vi "Test Event Registration.vi"() -> ()   [LabVIEW 2019]
panel:
  out "string 1":string
  in  "String Control":string
  in  "stop":bool
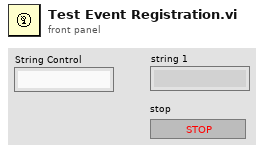
[diagram p1: front panel]
types:
  T1 = cluster{"string 2":refnum<user-event>, "string 3":refnum<user-event>}
  T2 = cluster{"Event Registration Refnum":refnum<event-registration>, "Event Registration Refnum":refnum<event-registration>}
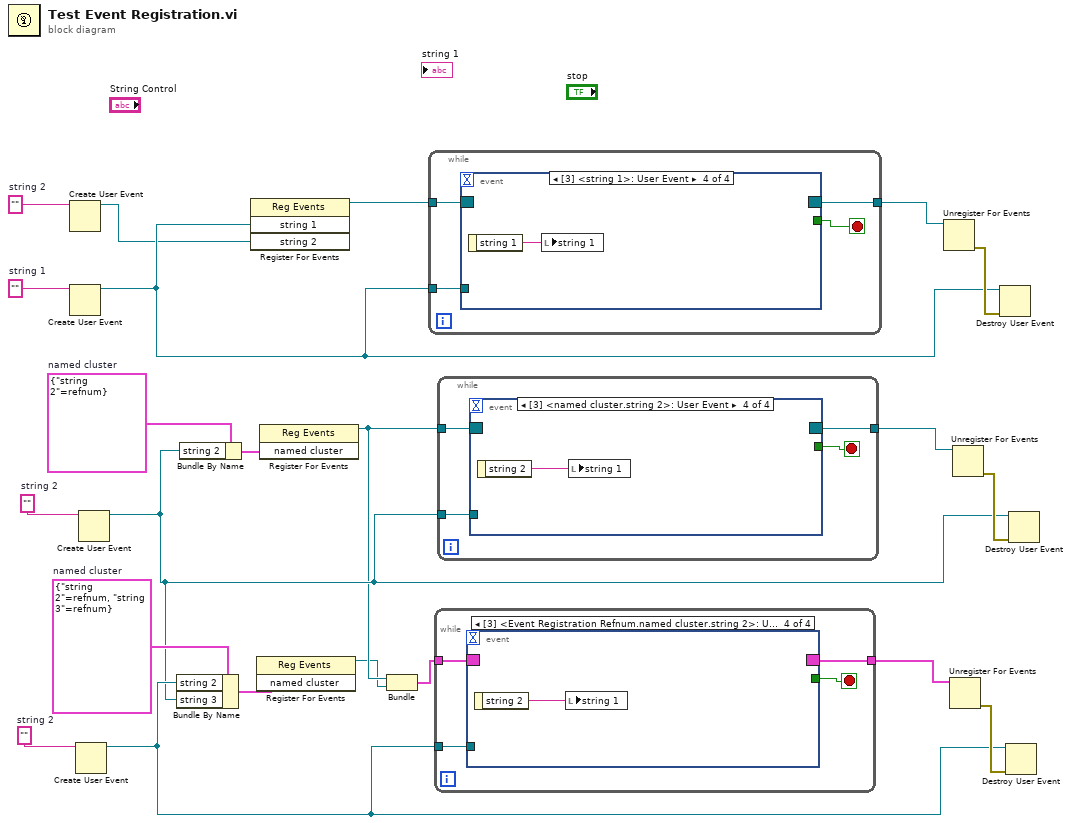
[diagram p0: block diagram]
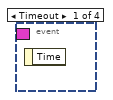
[diagram p2: hidden frame]
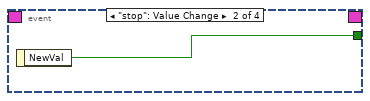
[diagram p3: hidden frame]
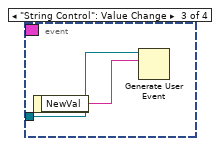
[diagram p4: hidden frame]
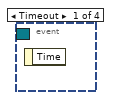
[diagram p5: hidden frame]
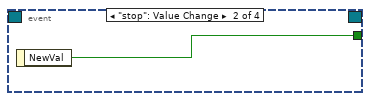
[diagram p6: hidden frame]
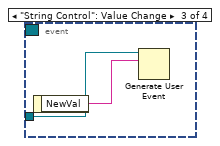
[diagram p7: hidden frame]
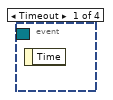
[diagram p8: hidden frame]
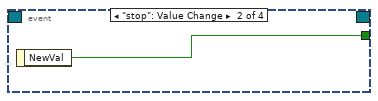
[diagram p9: hidden frame]
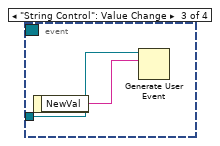
[diagram p10: hidden frame]
diagram:
  w5 = ""  # string 2
  w11 = T1 {"string 2"=refnum, "string 3"=refnum}  # named cluster
  w10 = ""  # string 2
  w14 = cluster{"string 2":refnum<user-event>} {"string 2"=refnum}  # named cluster
  w15 = ""  # string 2
  w21 = ""  # string 1
  n1 = Create User Event(user event datatype=w5) -> (user event=w4:refnum<user-event>)  [unwired: 1 in, 1 out]
  n2 = Create User Event(user event datatype=w21) -> (user event=w18:refnum<user-event>)  [unwired: 1 in, 1 out]
  n3 = Create User Event(user event datatype=w10) -> (user event=w7:refnum<user-event>)  [unwired: 1 in, 1 out]
  n4 = Create User Event(user event datatype=w15) -> (user event=w6:refnum<user-event>)  [unwired: 1 in, 1 out]
  n5 = Bundle By Name(cluster=w11, "string 2"=w7, "string 3"=w6) -> (w12:T1)
  n6 = Bundle By Name(cluster=w14, "string 2"=w6) -> (w13:cluster{"string 2":refnum<user-event>})
  n7 = register-events(w18, w4) -> (reference out=w22:refnum<event-registration>)  [unwired: 2 in, 1 out]
  n8 = register-events(w12) -> (reference out=w2:refnum<event-registration>)  [unwired: 2 in, 1 out]
  n9 = register-events(w13) -> (reference out=w3:refnum<event-registration>)  [unwired: 2 in, 1 out]
  n10 = Bundle("Event Registration Refnum"=w3, "Event Registration Refnum"=w2) -> (w1:T2)  [unwired: 1 in]
  n11 = while {
    tunnel: w22 -> [w25]
    tunnel: w18 -> [w24]
    tunnel: [w23] -> w20
    stop <- w26 stop-if-true
    n12 = event shown="[3] <string 1>: User Event" {
      selector: w25 -> [_ _ _ _]
      dyn-events: [_ _ _ _] -> w23
      timeout: _ -> [_ _ _ _]
      tunnel: [_ w27 _ _] -> w26
      tunnel: w24 -> [_ _ w29 _]
      event Timeout {
        n13 = event-data() -> ()  [unwired: 1 in, 1 out]
      }
      event "stop": Value Change {
        n14 = event-data() -> ("NewVal"=w27:bool)  [unwired: 1 in]
      }
      event "String Control": Value Change {
        n15 = event-data() -> ("NewVal"=w28:string)  [unwired: 1 in]
        n16 = Generate User Event(user event=w29, event data cluster=w28) -> ()  [unwired: 2 in, 2 out]
      }
      event User Event {
        n17 = event-data() -> ("string 1"=w30:string)  [unwired: 1 in]
        n18 = local write "string 1"(w30) -> ()
      }
    }
  }
  n19 = while {
    tunnel: w1 -> [w33]
    tunnel: w7 -> [w32]
    tunnel: [w31] -> w9
    stop <- w34 stop-if-true
    n20 = event shown="[3] <Event Registration Refnum.named cluster.string 2>: User Event" {
      selector: w33 -> [_ _ _ _]
      dyn-events: [_ _ _ _] -> w31
      timeout: _ -> [_ _ _ _]
      tunnel: [_ w35 _ _] -> w34
      tunnel: w32 -> [_ _ w37 _]
      event Timeout {
        n21 = event-data() -> ()  [unwired: 1 in, 1 out]
      }
      event "stop": Value Change {
        n22 = event-data() -> ("NewVal"=w35:bool)  [unwired: 1 in]
      }
      event "String Control": Value Change {
        n23 = event-data() -> ("NewVal"=w36:string)  [unwired: 1 in]
        n24 = Generate User Event(user event=w37, event data cluster=w36) -> ()  [unwired: 2 in, 2 out]
      }
      event User Event {
        n25 = event-data() -> ("string 2"=w38:string)  [unwired: 1 in]
        n26 = local write "string 1"(w38) -> ()
      }
    }
  }
  n27 = while {
    tunnel: w3 -> [w41]
    tunnel: w6 -> [w40]
    tunnel: [w39] -> w16
    stop <- w42 stop-if-true
    n28 = event shown="[3] <named cluster.string 2>: User Event" {
      selector: w41 -> [_ _ _ _]
      dyn-events: [_ _ _ _] -> w39
      timeout: _ -> [_ _ _ _]
      tunnel: [_ w43 _ _] -> w42
      tunnel: w40 -> [_ _ w45 _]
      event Timeout {
        n29 = event-data() -> ()  [unwired: 1 in, 1 out]
      }
      event "stop": Value Change {
        n30 = event-data() -> ("NewVal"=w43:bool)  [unwired: 1 in]
      }
      event "String Control": Value Change {
        n31 = event-data() -> ("NewVal"=w44:string)  [unwired: 1 in]
        n32 = Generate User Event(user event=w45, event data cluster=w44) -> ()  [unwired: 2 in, 2 out]
      }
      event User Event {
        n33 = event-data() -> ("string 2"=w46:string)  [unwired: 1 in]
        n34 = local write "string 1"(w46) -> ()
      }
    }
  }
  n35 = Unregister For Events(event registration refnum=w20) -> (error out=w19:errorcluster)  [unwired: 1 in]
  n36 = Unregister For Events(event registration refnum=w9) -> (error out=w8:errorcluster)  [unwired: 1 in]
  n37 = Unregister For Events(event registration refnum=w16) -> (error out=w17:errorcluster)  [unwired: 1 in]
  n38 = Destroy User Event(user event=w18, error in=w19) -> ()  [unwired: 1 out]
  n39 = Destroy User Event(user event=w7, error in=w8) -> ()  [unwired: 1 out]
  n40 = Destroy User Event(user event=w6, error in=w17) -> ()  [unwired: 1 out]
